vi "Write Watchdog Config.vi"() -> (0 "error out":errorcluster)   [LabVIEW 2020]
panel:
  out "Error String":string
  out "ConnectionType Out":i32
  out "DeviceType Out":i32
  in  "Identifier":string="LJM_idANY"
  in  "ConnectionType":string="LJM_ctANY"
  in  "DeviceType":string="LJM_dtANY"
  in  "Values":dbl[](array[numeric])=[0.0, 0.0, 10.0, 0.0, 0.0, 0.0, 1.0, 0.0, 0.0, 0.0, 0.0, 0.0, 0.0, 0.0, 0.0, 0.0] format="%.2f"
  in  "Names":string[](array[string])=["WATCHDOG_ENABLE_DEFAULT", "WATCHDOG_ADVANCED_DEFAULT", "WATCHDOG_TIMEOUT_S_DEFAULT", "WATCHDOG_STARTUP_DELAY_S_DEFAULT", "WATCHDOG_STRICT_ENABLE_DEFAULT", "WATCHDOG_STRICT_KEY_DEFAULT", "WATCHDOG_RESET_ENABLE_DEFAULT", "WATCHDOG_DIO_ENABLE_DEFAULT", "WATCHDOG_DIO_STATE_DEFAULT", "WATCHDOG_DIO_DIRECTION_DEFAULT", "WATCHDOG_DIO_INHIBIT_DEFAULT", "WATCHDOG_DAC0_ENABLE_DEFAULT", "WATCHDOG_DAC0_DEFAULT", "WATCHDOG_DAC1_ENABLE_DEFAULT", "WATCHDOG_DAC1_DEFAULT", "WATCHDOG_ENABLE_DEFAULT"]
  out "ErrorAddress":i32
  # "<-- Set to 1 to enable the watchdog."
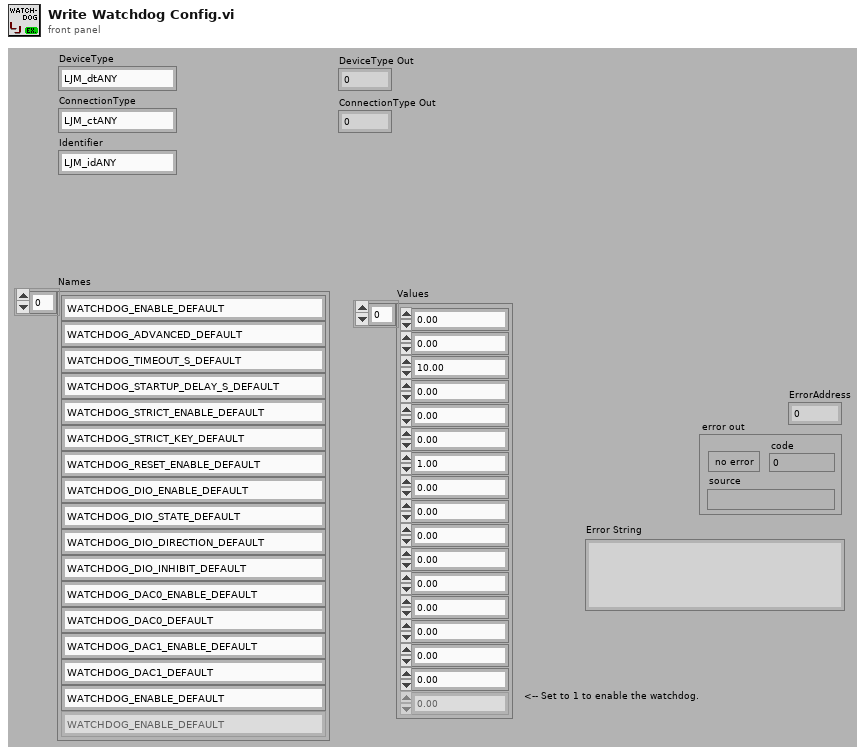
[diagram p1: front panel]
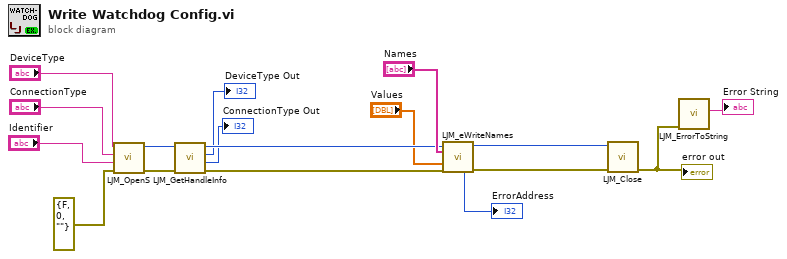
[diagram p0: block diagram]
diagram:
  n1 = call "LJM_OpenS.vi"("error in"=errorcluster {"status"=FALSE, "code"=0, "source"=""} ("error in (no error)"), "Identifier"="Identifier", "ConnectionType"="ConnectionType", "DeviceType"="DeviceType") -> ("error out"=w14:errorcluster, "Handle"=w12:i32)  [unwired: 6 in]
  n2 = call "LJM_GetHandleInfo.vi"("error in"=w14, "Handle In"=w12) -> ("error out"=w13:errorcluster, "ConnectionType"=→"ConnectionType Out":i32, "DeviceType"=→"DeviceType Out":i32, "Handle Out"=w11:i32)  [unwired: 2 in, 4 out]
  n3 = call "LJM_eWriteNames.vi"("Handle In"=w11, "aNames"="Names", "aValuesIn"="Values", "error in"=w13) -> ("Handle Out"=w10:i32, "ErrorAddress"=→"ErrorAddress":i32, "error out"=w16:errorcluster)  [unwired: 9 in]
  n4 = call "LJM_Close.vi"("error in"=w16, "Handle"=w10) -> ("error out"=w4:errorcluster)  [unwired: 9 in]
  "error out" <- w4
  n5 = call "LJM_ErrorToString.vi"("error in"=w4) -> ("String"=→"Error String":string)  [unwired: 10 in]
